vi "Connection.vi"() -> ()   [LabVIEW 2013]
uses:
  <userlib>/GCSLabView/Low Level/Communication.llb/Available interfaces.ctl
panel:
  out "Conn. Axes out":string[](array[string])
  out "error out":errorcluster
  in  "Flow control":T1={"input XON/XOFF"=FALSE, "input HW Handshake"=FALSE, "input alt HW HShk"=FALSE, "output XON/XOFF"=FALSE, "output HW Handshake"=FALSE, "output alt HW HShk"=FALSE, "XOFF byte "=19, "XON byte"=17, "parity error byte"=0} {"parity error byte" format="%.0x"; "XON byte" format="%.0x"; "XOFF byte" format="%.0x"}
  out "Position":dbl[](array[numeric]) format="%.6f"
  in  "Bit settings and parity":T2={"data bits"=8, "stop bits"=enum."1 bit", "parity"=enum."no parity"} {"data bits" min=5 max=8 step=1}
  in  "Interface configuration":T4={"RS232 Portnumber"=2, "Timeout"=500, "RS232 Baud rate"=38400, "Interface"=0, "GPIB Bus"=0, "GPIB Address"=4, "GPIB Mode"=0} {"RS232 Portnumber" items=["COM1", "COM2", "COM3", "COM4", "COM5", "COM6", "COM7", "COM8", "COM9", "COM10", "COM11", "COM12", "COM13", "COM14", "COM15", "COM16", "COM17", "COM18", "COM19", "COM20", "COM21", "COM22", "COM23", "COM24", "COM25", "COM26", "COM27", "COM28", "COM29", "COM30"]; "Interface" items=["RS232", "GPIB", "DLL", "TCP-IP", "USB", "Analog"]}
  out "Identification":string
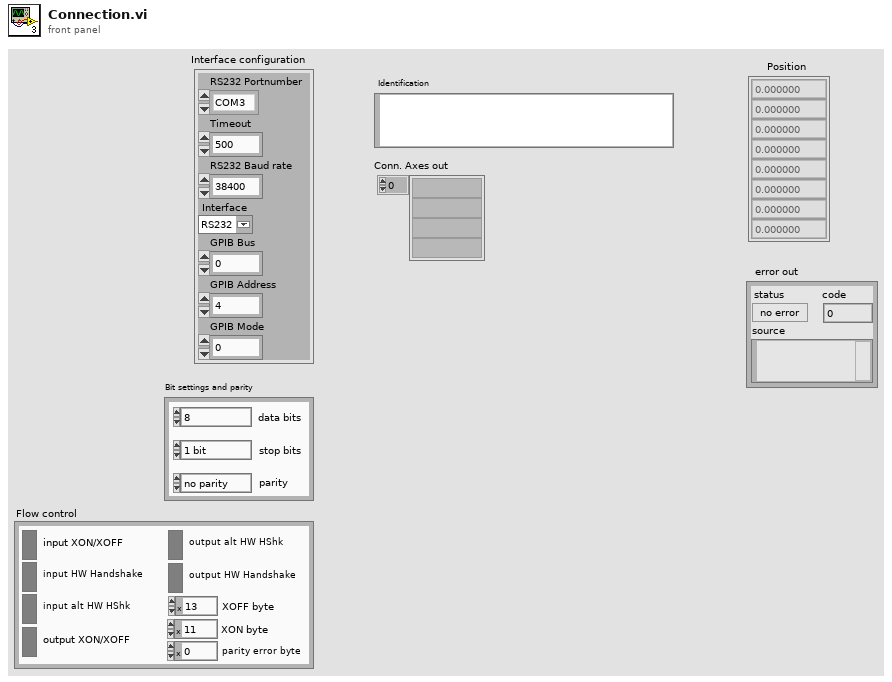
[diagram p1: front panel]
types:
  T1 = cluster{"input XON/XOFF":bool, "input HW Handshake":bool, "input alt HW HShk":bool, "output XON/XOFF":bool, "output HW Handshake":bool, "output alt HW HShk":bool, "XOFF byte ":u8, "XON byte":u8, "parity error byte":u16}
  T2 = cluster{"data bits":u16, "stop bits":enum16{"1 bit", "1.5 bits", "2 bits"}, "parity":enum16{"no parity", "odd parity", "even parity", "mark parity", "space parity"}}
  T3 = typedef "Available interfaces.ctl" = u16
  T4 = cluster{"RS232 Portnumber":i32, "Timeout":i32, "RS232 Baud rate":u32, "Interface":T3, "GPIB Bus":i32, "GPIB Address":i32, "GPIB Mode":i32}
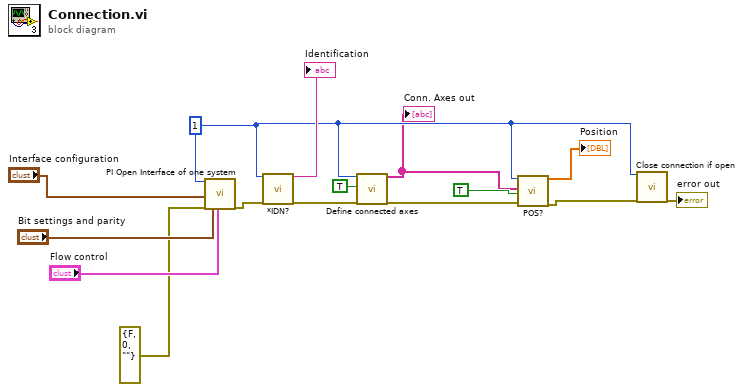
[diagram p0: block diagram]
diagram:
  w4 = 1 ("System number")
  n1 = call <userlib>:"PI Open Interface of one system.vi"("System number"=w4, "Interface configuration"="Interface configuration", "error in"=errorcluster {"status"=FALSE, "code"=0, "source"=""}, "Bit settings and parity"="Bit settings and parity", "Flow control"="Flow control") -> ("error out"=w14:errorcluster)  [unwired: 13 in, 1 out]
  n2 = call <userlib>:"*IDN?.vi"("System no."=w4, "error in"=w14) -> ("Identification"=→"Identification":string, "error out"=w5:errorcluster)  [unwired: 16 in]
  n3 = call <userlib>:"Define connected axes.vi"("System no."=w4, "Read from\ncontroller?"=TRUE ("Read from\ncontroller?"), "error in"=w5) -> ("Conn. Axes out"=w3:string[], "error out"=w2:errorcluster)  [unwired: 15 in]
  "Conn. Axes out" <- w3
  n4 = call <userlib>:"POS?.vi"("System no."=w4, "Axes to query"=w3, "All axes?"=TRUE, "error in"=w2) -> ("Position"=→"Position":dbl[], "error out"=w9:errorcluster)  [unwired: 14 in]
  n5 = call <userlib>:"Close connection if open.vi"("System no."=w4, "error in"=w9) -> ("error out"=→"error out":errorcluster)  [unwired: 16 in, 1 out]
